vi "Execute.vi"(8 "error in (no error)":errorcluster, 11 "Node in":refnum<class "Measure Waveform.lvclass">) -> (0 "error out":errorcluster, 1 "Status":T1, 3 "Node out":refnum<class "Measure Waveform.lvclass">)   [LabVIEW 2021, in "Measure Waveform.lvclass"]
uses:
  Measure Waveform.lvclass
  Support/Nodes/abs_Node/Status.ctl
  Measure Waveform.lvclass/Measure Waveform.ctl
  <vilib>/TSA/Abstract Data Classes/Abs_Types/Waveform/Static Read.vi
  <vilib>/TSA/Abstract Data Classes/Abs_Types/Double Float/Static Write.vi
  Properties/Read Abs_Waveform.vi
  Properties/Read Measured Phase.vi
  Properties/Read Measured Amplitude.vi
  Properties/Read Measured Frequency.vi
  <vilib>/measure/matone.llb/Extract Single Tone Information 1 Chan.vi
  <vilib>/TSA/Abstract Data Classes/Abs_Types/Waveform/Abs_Waveform.lvclass
  <vilib>/TSA/Abstract Data Classes/Abs_Types/Double Float/Abs_Double Float.lvclass
  <vilib>/measure/NI_MAPro.lvlib
  Support/Nodes/abs_Node/bt_Node.lvclass
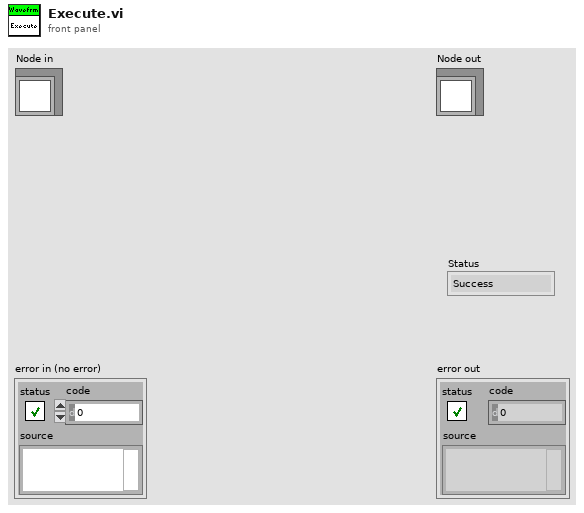
[diagram p1: front panel]
types:
  T1 = typedef "BT.lvlib/bt_Node.lvclass/Status.ctl" = enum16{"Success", "Failure", "Running"}
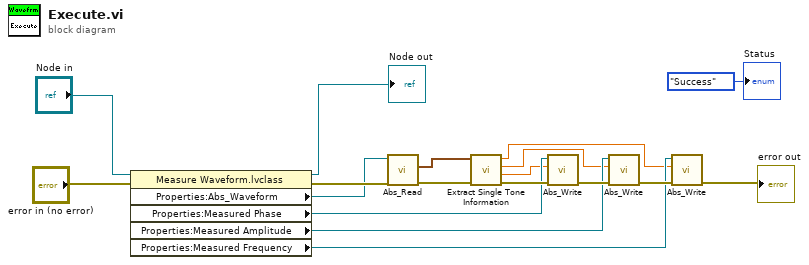
[diagram p0: block diagram]
diagram:
  n1 = property class="Measure Waveform.lvclass"(reference="Node in", error in="error in (no error)") -> (reference out=→"Node out":refnum<class "Measure Waveform.lvclass">, error out=w16:errorcluster, "Properties:Abs_Waveform"=w15:refnum<class "Abs_Waveform.lvclass">, "Properties:Measured Phase"=w8:refnum<class "Abs_Double Float.lvclass">, "Properties:Measured Amplitude"=w7:refnum<class "Abs_Double Float.lvclass">, "Properties:Measured Frequency"=w6:refnum<class "Abs_Double Float.lvclass">)
  n2 = call-poly <vilib>:"Abs_Read.vi"("error in (no error)"=w16, "Abs_Waveform in"=w15) -> ("error out"=w14:errorcluster, "Waveform"=w13:waveform(dbl))  [unwired: 7 in, 1 out]
  n3 = call-poly <vilib>:"Extract Single Tone Information.vi"("error in (no error)"=w14, "time signal in"=w13) -> ("error out"=w11:errorcluster, "detected phase (deg)"=w3:dbl, "detected amplitude"=w2:dbl, "detected frequency"=w1:dbl)  [unwired: 4 in, 2 out]
  n4 = call-poly <vilib>:"Abs_Write.vi"("error in (no error)"=w11, "Value"=w3, "Abs_Double Float in"=w8) -> ("error out"=w10:errorcluster)  [unwired: 7 in, 1 out]
  n5 = call-poly <vilib>:"Abs_Write.vi"("error in (no error)"=w10, "Value"=w2, "Abs_Double Float in"=w7) -> ("error out"=w9:errorcluster)  [unwired: 7 in, 1 out]
  n6 = call-poly <vilib>:"Abs_Write.vi"("error in (no error)"=w9, "Value"=w1, "Abs_Double Float in"=w6) -> ("error out"=→"error out":errorcluster)  [unwired: 7 in, 1 out]
  "Status" <- Status."Success" ("Status")
